vi "Pack Data.vi"(5 "Math":T3, 6 "Encoder":T2) -> (0 "RR Data":T1, 1 "RL Data":T1, 2 "FL Data":T1, 3 "FR Data":T1)   [LabVIEW 2018]
uses:
  Motor Data Unpacked.ctl
  Encoder Unpacked Data.ctl
  Final Motor Data.ctl
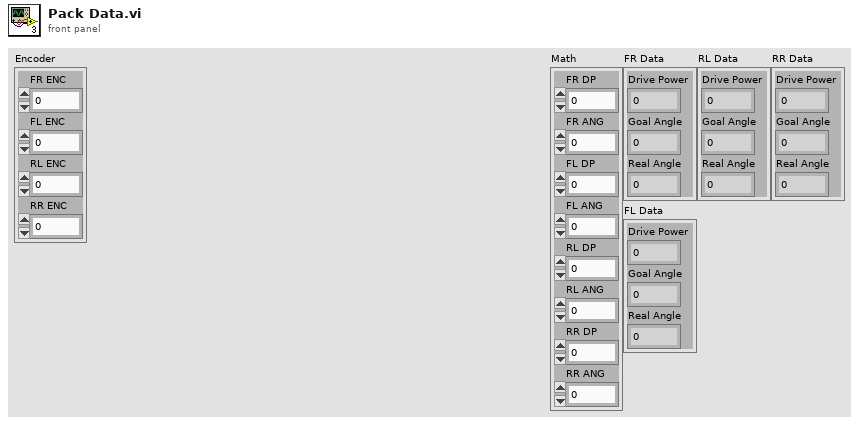
[diagram p1: front panel]
types:
  T1 = typedef "Final Motor Data.ctl" = cluster{"Drive Power":dbl, "Goal Angle":dbl, "Real Angle":dbl}
  T2 = typedef "Encoder Unpacked Data.ctl" = cluster{"FR ENC":dbl, "FL ENC":dbl, "RL ENC":dbl, "RR ENC":dbl}
  T3 = typedef "Motor Data Unpacked.ctl" = cluster{"FR DP":dbl, "FR ANG":dbl, "FL DP":dbl, "FL ANG":dbl, "RL DP":dbl, "RL ANG":dbl, "RR DP":dbl, "RR ANG":dbl}
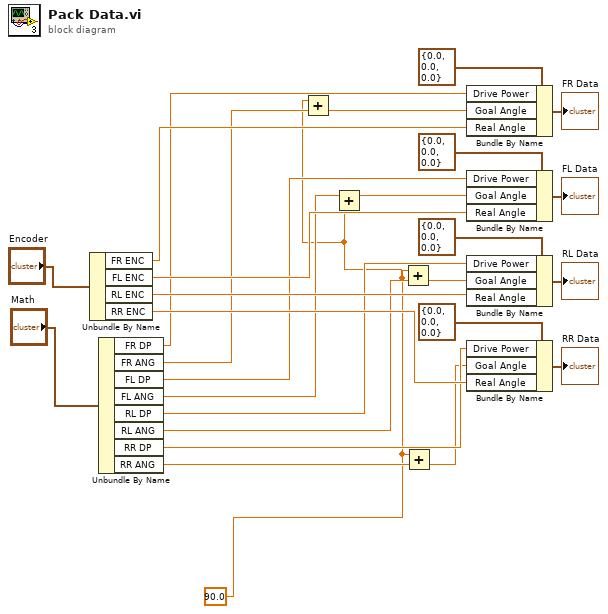
[diagram p0: block diagram]
diagram:
  w1 = 90.0
  n1 = Unbundle By Name("Encoder") -> ("FR ENC"=w21:dbl, "FL ENC"=w20:dbl, "RL ENC"=w19:dbl, "RR ENC"=w18:dbl)
  n2 = Unbundle By Name("Math") -> ("FR DP"=w17:dbl, "FR ANG"=w15:dbl, "FL DP"=w16:dbl, "FL ANG"=w14:dbl, "RL DP"=w13:dbl, "RL ANG"=w12:dbl, "RR DP"=w11:dbl, "RR ANG"=w10:dbl)
  n3 = Add(x=w1, y=w15) -> (x+y=w5:dbl)
  n4 = Add(x=w14, y=w1) -> (x+y=w4:dbl)
  n5 = Add(x=w1, y=w12) -> (x+y=w3:dbl)
  n6 = Add(x=w1, y=w10) -> (x+y=w2:dbl)
  n7 = Bundle By Name(cluster=T1 {"Drive Power"=0.0, "Goal Angle"=0.0, "Real Angle"=0.0}, "Drive Power"=w17, "Goal Angle"=w5, "Real Angle"=w21) -> (→"FR Data":T1)
  n8 = Bundle By Name(cluster=T1 {"Drive Power"=0.0, "Goal Angle"=0.0, "Real Angle"=0.0}, "Drive Power"=w16, "Goal Angle"=w4, "Real Angle"=w20) -> (→"FL Data":T1)
  n9 = Bundle By Name(cluster=T1 {"Drive Power"=0.0, "Goal Angle"=0.0, "Real Angle"=0.0}, "Drive Power"=w13, "Goal Angle"=w3, "Real Angle"=w19) -> (→"RL Data":T1)
  n10 = Bundle By Name(cluster=T1 {"Drive Power"=0.0, "Goal Angle"=0.0, "Real Angle"=0.0}, "Drive Power"=w11, "Goal Angle"=w2, "Real Angle"=w18) -> (→"RR Data":T1)
